vi "Write Acceleration.vi"(8 "error in (no error)":errorcluster, 10 "Acceleration":T1, 11 "XY Stage Data Class in":refnum<class "XY Stage Data Class.lvclass">) -> (0 "error out":errorcluster, 3 "XY Stage Data Class out":refnum<class "XY Stage Data Class.lvclass">)   [LabVIEW 2022 SP3, in "XY Stage Data Class.lvclass"]
uses:
  XY Stage Data Class.lvclass
  Acceleration.ctl
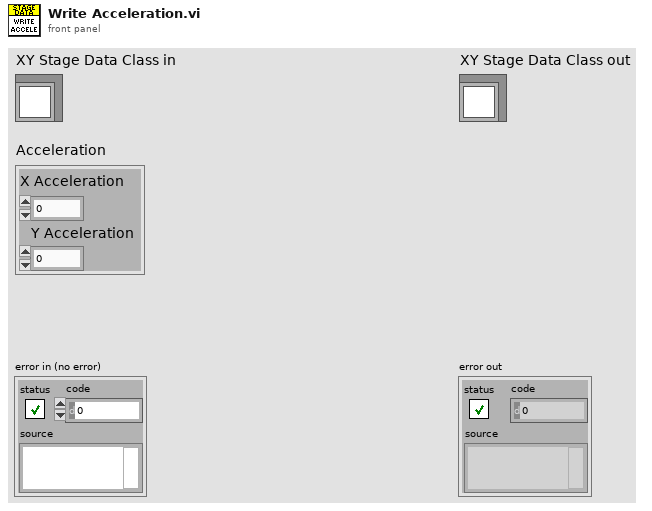
[diagram p1: front panel]
types:
  T1 = typedef "XY Stage Data Class.lvclass/Acceleration.ctl" = cluster{"X Acceleration":dbl, "Y Acceleration":dbl}
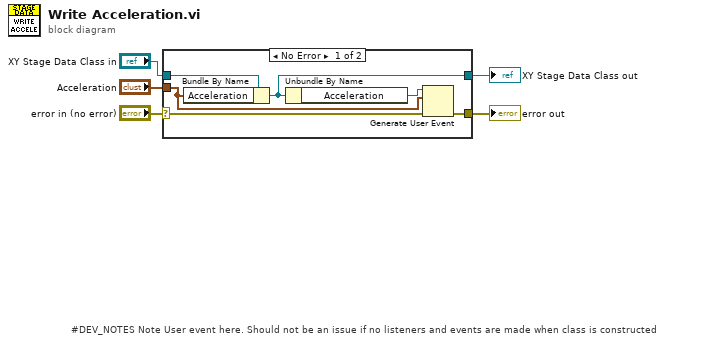
[diagram p0: block diagram]
diagram:
  # "#DEV_NOTES Note User event here. Should not be an issue if no listeners and events are made when class is constructed"
  n1 = case shown="No Error" "error in (no error)" {
    selector: "error in (no error)" -> [w7 w12]
    tunnel: [w6 w12] -> w4
    tunnel: [w10 w13] -> w2
    tunnel: "XY Stage Data Class in" -> [w11 w13]
    tunnel: "Acceleration" -> [w8 _]
    frame No Error {
      n2 = Bundle By Name(cluster=w11, "Acceleration"=w8) -> (w10:refnum<class "XY Stage Data Class.lvclass">)
      n3 = Unbundle By Name(w10) -> ("Acceleration"=w9:refnum<user-event>)
      n4 = Generate User Event(user event=w9, event data cluster=w8, error in=w7) -> (error out=w6:errorcluster)  [unwired: 1 in, 1 out]
    }
    frame Error {
    }
  }
  "error out" <- w4
  "XY Stage Data Class out" <- w2
